vi "PowerSpectrumTest.vi"() -> ()   [LabVIEW 2012]
uses:
  <vilib>/Analysis/NI_AALBase.lvlib
  <vilib>/Analysis/NI_AALPro.lvlib
panel:
  out "PercentageDifference LV":dbl
  out "PercentageDifference EnFlo":dbl
  out "Old-new":dbl format="%_6e"
  out "E(f).dF LV":dbl
  out "E(f).dF Old":dbl
  out "E(f).dF New":dbl
  out "Signal variance":dbl format="%.6f"
  in  "amplitude":dbl=1.0 format="%0.2f"
  in  "samples":i32=128
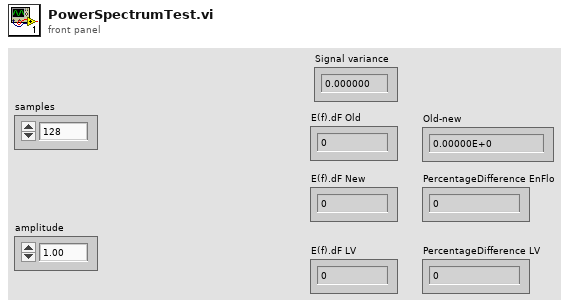
[diagram p1: front panel]
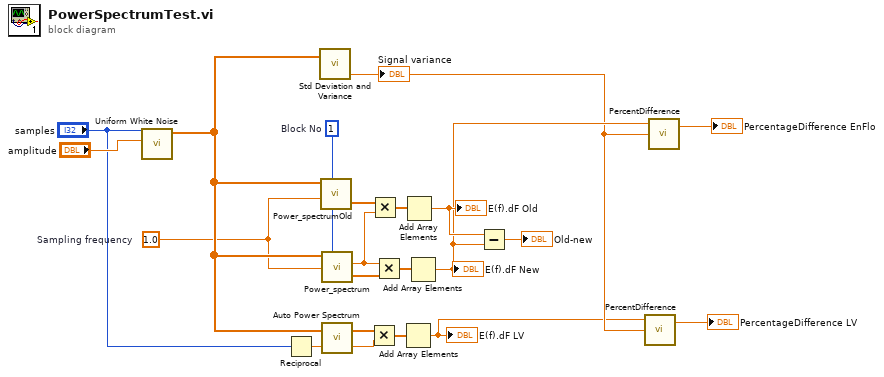
[diagram p0: block diagram]
diagram:
  w2 = sgl 1.0  # Sampling frequency
  w20 = 1  # Block No
  n1 = call <vilib>:"Uniform White Noise.vi"("amplitude"="amplitude", "samples"="samples") -> ("uniform white noise"=w3:dbl[])  [unwired: 8 in, 1 out]
  n2 = Reciprocal(x="samples") -> (1/x=w13:dbl)
  n3 = call <vilib>:"Std Deviation and Variance.vi"("X"=w3) -> ("variance"=w5:dbl)  [unwired: 1 in, 2 out]
  "Signal variance" <- w5
  n4 = call "Power_spectrumOld.vi"("U"=w3, "Sampling frequency"=w2, "Block No"=w20) -> ("Spectrum output array"=w16:dbl[])  [unwired: 3 in]
  n5 = call "Power_spectrum.vi"("U"=w3, "Sampling frequency"=w2, "Block No"=w20) -> ("dF"=w15:dbl, "Spectrum output array"=w19:dbl[])  [unwired: 2 in]
  n6 = call <vilib>:"Auto Power Spectrum.vi"("dt"=w13, "Signal (V)"=w3) -> ("df"=w11:dbl, "Power Spectrum (V^2 rms)"=w12:dbl[])
  n7 = Multiply(x=w12, y=w11) -> (x*y=w14:dbl[])
  n8 = Multiply(x=w16, y=w15) -> (x*y=w17:dbl[])
  n9 = Multiply(x=w15, y=w19) -> (x*y=w18:dbl[])
  n10 = Add Array Elements(numeric array=w14) -> (sum=w4:dbl)
  "E(f).dF LV" <- w4
  n11 = Add Array Elements(numeric array=w17) -> (sum=w10:dbl)
  "E(f).dF Old" <- w10
  n12 = Add Array Elements(numeric array=w18) -> (sum=w8:dbl)
  "E(f).dF New" <- w8
  n13 = Subtract(x=w10, y=w8) -> (x-y=→"Old-new":dbl)
  n14 = call "PercentDifference.vi"("Basis"=w5, "Comparee"=w4) -> ("PercentageDifference"=→"PercentageDifference LV":dbl)  [unwired: 1 in, 1 out]
  n15 = call "PercentDifference.vi"("Basis"=w5, "Comparee"=w8) -> ("PercentageDifference"=→"PercentageDifference EnFlo":dbl)  [unwired: 1 in, 1 out]
